vi "[Generate Test Cases] Put and Get file.vi"(11 "Targets":T1(array[cluster])) -> (3 "Test Cases":refnum<class "TestCase.lvclass">[](array[class]))   [LabVIEW 2015, in "Tests.lvlib" / "[Test Suite] File Transfer Behavior.lvclass"]
uses:
  [Test Suite] File Transfer Behavior.lvclass
  <vilib>/addons/_JKI Toolkits/VI Tester/TestCase.llb/TestCase.lvclass
  classes/FTP/FTP.lvclass
  classes/WebDAV/WebDAV.lvclass
  classes/File Transfer Behavior/File Transfer Behavior.lvclass
  classes/File Transfer Behavior/File Transfer Behavior.lvclass/File Transfer Behavior.ctl
  [Test Case] Put and Get file/[Test Case] Put and Get file.lvclass
  [Test Case] Put and Get file/[Test Case] Put and Get file.lvclass/[Test Case] Put and Get file.ctl
  [Test Case] Put and Get file/Write File Transfer Behavior.lvclass.vi
  [Test Case] Put and Get file/Write Local path.vi
  [Test Case] Put and Get file/Write Remote path.vi
  classes/File Transfer Behavior/Set Address.vi
  classes/File Transfer Behavior/Set Password.vi
  classes/File Transfer Behavior/Set Username.vi
  Tests.lvlib
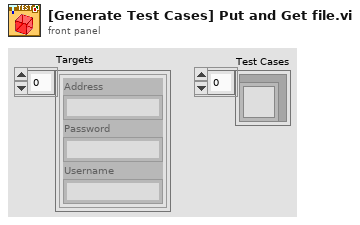
[diagram p1: front panel]
types:
  T1 = cluster{"Address":string, "Password":string, "Username":string}[]
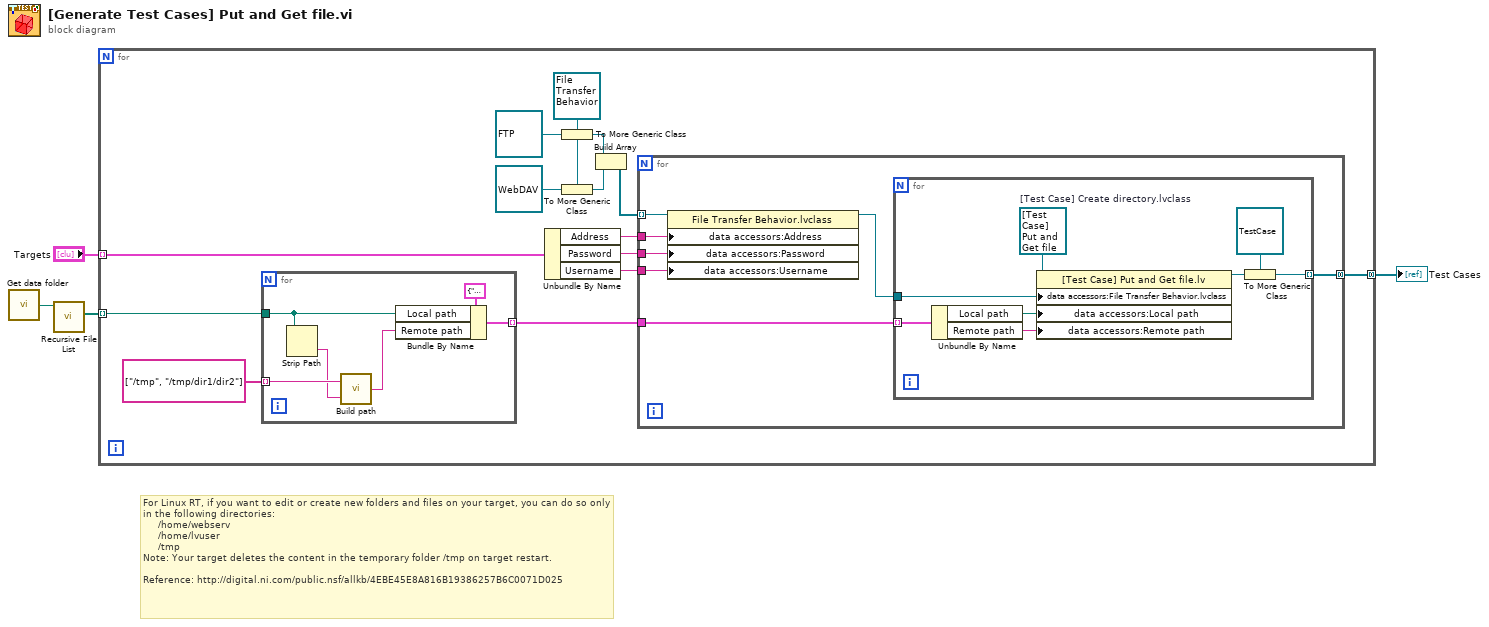
[diagram p0: block diagram]
diagram:
  # "For Linux RT, if you want to edit or create new folders and files on your target, you can do so only in the following directories:\n     /home/webserv\n     /home/lvuser\n     /tmp\nNote: Your target deletes the content in the temporary folder /tmp on target restart.\n\nReference: http://digital.ni.com/public.nsf/allkb/4EBE45E8A816B19386257B6C0071D025"
  n1 = call "Get data folder.vi"() -> ("Data folder"=w2:path)
  n2 = call <vilib>:"Recursive File List.vi"("Folder Path"=w2) -> ("All Files in Dir"=w1:path[])  [unwired: 6 in, 4 out]
  n3 = for {
    tunnel: [w18] -> w4 mode=concatenating
    tunnel: "Targets" -> [w14] mode=indexing
    tunnel: w1 -> [w7] mode=indexing
    w13 = refnum<class "File Transfer Behavior.lvclass"> refnum ("RT Management.lvlib:File Transfer Behavior.lvclass")
    n4 = for {
      tunnel: w7 -> [w23]
      tunnel: string[] ["/tmp", "/tmp/dir1/dir2"] -> [w22] mode=indexing
      tunnel: [w19] -> w5 mode=indexing
      n5 = Strip Path(path=w23) -> (name=w21:string)  [unwired: 1 out]
      n6 = call "Build path.vi"("Relative path"=w21, "Base path"=w22) -> ("Resulting path"=w20:string)
      n7 = Bundle By Name(cluster=cluster{"Remote path":string, "Local path":path} {"Remote path"="", "Local path"=path ""}, "Local path"=w23, "Remote path"=w20) -> (w19:cluster{"Remote path":string, "Local path":path})
    }
    n8 = Unbundle By Name(w14) -> ("Address"=w17:string, "Password"=w16:string, "Username"=w15:string)
    n9 = To More Generic Class(target class=w13, reference=refnum<class "FTP.lvclass"> refnum ("RT Management.lvlib:FTP.lvclass")) -> (generic class reference=w10:refnum<class "File Transfer Behavior.lvclass">)
    n10 = To More Generic Class(target class=w13, reference=refnum<class "WebDAV.lvclass"> refnum ("RT Management.lvlib:WebDAV.lvclass")) -> (generic class reference=w9:refnum<class "File Transfer Behavior.lvclass">)
    n11 = Build Array(w10, w9) -> (w8:refnum<class "File Transfer Behavior.lvclass">[])
    n12 = for {
      tunnel: w17 -> [w30]
      tunnel: w16 -> [w29]
      tunnel: w15 -> [w28]
      tunnel: [w27] -> w18 mode=concatenating
      tunnel: w8 -> [w26] mode=indexing
      tunnel: w5 -> [w25]
      n13 = property class="File Transfer Behavior.lvclass"(reference=w26, "data accessors:Address"=w30, "data accessors:Password"=w29, "data accessors:Username"=w28) -> (reference out=w31:refnum<class "File Transfer Behavior.lvclass">)  [unwired: 1 in, 1 out]
      n14 = for {
        tunnel: w31 -> [w38]
        tunnel: [w35] -> w27 mode=indexing
        tunnel: w25 -> [w34] mode=indexing
        w39 = refnum<class "[Test Case] Put and Get file.lvclass"> refnum  # [Test Case] Create directory.lvclass
        n15 = Unbundle By Name(w34) -> ("Local path"=w32:path, "Remote path"=w33:string)
        n16 = property class="[Test Case] Put and Get file.lv"(reference=w39, "data accessors:File Transfer Behavior.lvclass"=w38, "data accessors:Local path"=w32, "data accessors:Remote path"=w33) -> (reference out=w37:refnum<class "[Test Case] Put and Get file.lvclass">)  [unwired: 1 in, 1 out]
        n17 = To More Generic Class(target class=refnum<class "TestCase.lvclass"> refnum ("TestCase.lvclass"), reference=w37) -> (generic class reference=w35:refnum<class "TestCase.lvclass">)
      }
    }
  }
  "Test Cases" <- w4
